vi "IsAdmin.vi"(8 "Error In":errorcluster) -> (0 "Error Out":errorcluster, 3 "Is Admin?":bool)   [LabVIEW 2019, in "CEPM.lvlib"]
uses:
  CEPM.lvlib
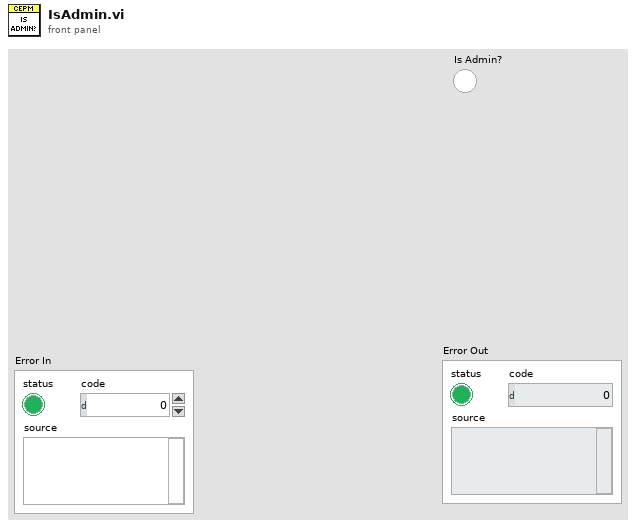
[diagram p1: front panel]
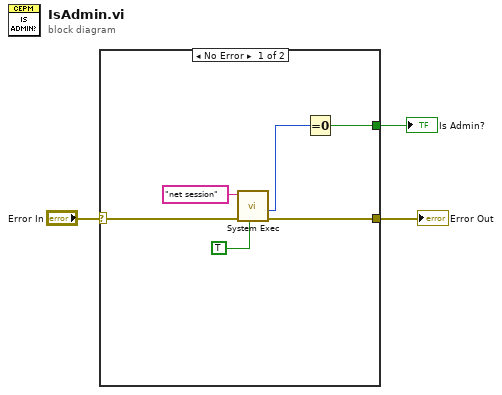
[diagram p0: block diagram]
diagram:
  n1 = case shown="No Error" "Error In" {
    selector: "Error In" -> [w9 w10]
    tunnel: [w8 w10] -> w2
    tunnel: [w4 _] -> w1
    frame No Error {
      n2 = call <vilib>:"System Exec.vi"("run minimized? (F)"=TRUE, "error in (no error)"=w9, "command line"="net session") -> ("error out"=w8:errorcluster, "return code"=w5:i32)  [unwired: 5 in, 2 out]
      n3 = Equal To 0?(x=w5) -> (x = 0?=w4:bool)
    }
    frame Error {
    }
  }
  "Error Out" <- w2
  "Is Admin?" <- w1
